vi "addRegExElement.vi"(6 "options":T1, 7 "Name":string, 8 "error in (no error)":errorcluster, 9 "Regular Expression":string, 10 "Replace? (false)":bool, 11 "tBSONDocument in":refnum<class "tBSONDocument.lvclass">) -> (0 "error out":errorcluster, 3 "tBSONDocument out":refnum<class "tBSONDocument.lvclass">)   [LabVIEW 2013, in "BSON.lvlib" / "tBSONDocument.lvclass"]
doc: "Adds a regular expression to a BSON document."
uses:
  tBSONDocument.lvclass
  BSONElements/tBSONRegEx/options.ctl
  BSONElements/tBSONRegEx/tBSONRegEx.lvclass
  tBSONElement/tBSONElement.lvclass
  tBSONElement/setName.vi
  BSONElements/tBSONRegEx/setRegularExpression.vi
  BSONElements/tBSONRegEx/setOptions.vi
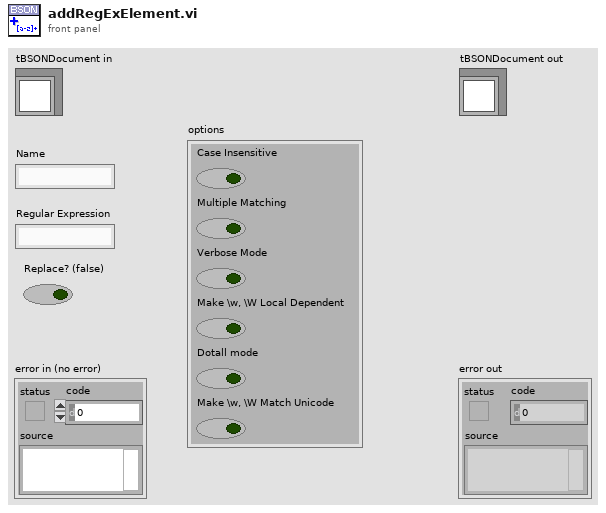
[diagram p1: front panel]
types:
  T1 = typedef "BSON.lvlib/tBSONRegEx.lvclass/options.ctl" = cluster{"Case Insensitive":bool, "Multiple Matching":bool, "Verbose Mode":bool, "Make \\w, \\W Local Dependent":bool, "Dotall mode":bool, "Make \\w, \\W Match Unicode":bool}
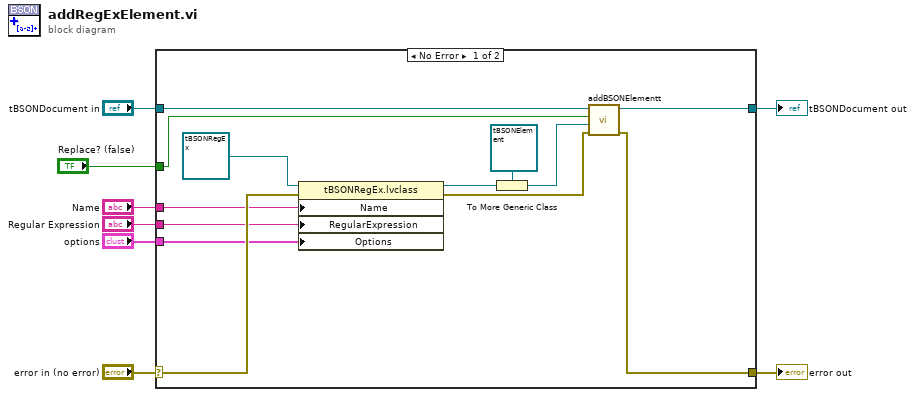
[diagram p0: block diagram]
diagram:
  n1 = case shown="No Error" "error in (no error)" {
    selector: "error in (no error)" -> [w20 w23]
    tunnel: [w10 w23] -> w7
    tunnel: [w18 w22] -> w5
    tunnel: "tBSONDocument in" -> [w19 w22]
    tunnel: "Name" -> [w13 _]
    tunnel: "Regular Expression" -> [w12 _]
    tunnel: "options" -> [w11 _]
    tunnel: "Replace? (false)" -> [w9 _]
    frame No Error {
      n2 = property class="tBSONRegEx.lvclass"(reference=refnum<class "tBSONRegEx.lvclass"> refnum ("BSON.lvlib:tBSONRegEx.lvclass"), error in=w20, "Name"=w13, "RegularExpression"=w12, "Options"=w11) -> (reference out=w15:refnum<class "tBSONRegEx.lvclass">, error out=w17:errorcluster)
      n3 = To More Generic Class(target class=refnum<class "tBSONElement.lvclass"> refnum ("BSON.lvlib:tBSONElement.lvclass"), reference=w15) -> (generic class reference=w14:refnum<class "tBSONElement.lvclass">)
      n4 = call "addBSONElementt.vi"("error in (no error)"=w17, "Element"=w14, "Replace? (false)"=w9, "tBSONDocument in"=w19) -> ("error out"=w10:errorcluster, "tBSONDocument out"=w18:refnum<class "tBSONDocument.lvclass">)  [unwired: 6 in]
    }
    frame Error {
    }
  }
  "error out" <- w7
  "tBSONDocument out" <- w5
